vi "删除启动项.vi"(8 "error in (no error)":errorcluster caption="错误输入（无错误）") -> (0 "error out":errorcluster caption="错误输出", 3 "删除标记":bool)   [LabVIEW 2016]
uses:
  <vilib>/registry/registry.llb/Registry RtKey.ctl
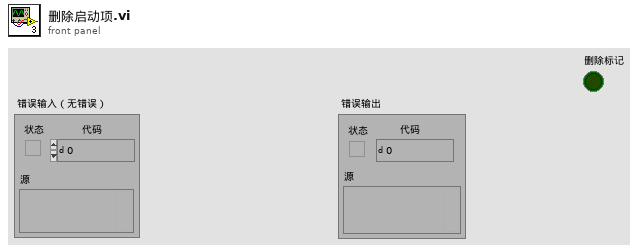
[diagram p1: front panel]
types:
  T1 = typedef "Registry RtKey.ctl" = enum32{"HKEY_CLASSES_ROOT", "HKEY_CURRENT_USER", "HKEY_LOCAL_MACHINE", "HKEY_USERS", "HKEY_PERFORMANCE_DATA", "HKEY_CURRENT_CONFIG", "HKEY_DYN_DATA"}
  T2 = typedef "Registry refnum.ctl" = refnum<k1>
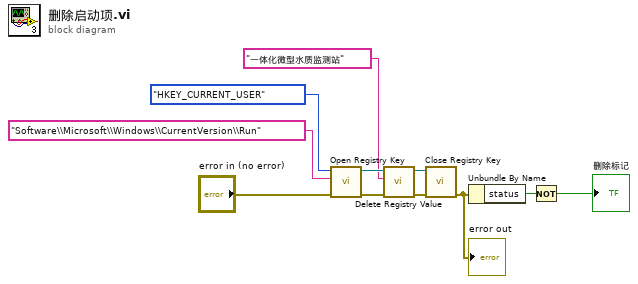
[diagram p0: block diagram]
diagram:
  n1 = call <vilib>:"Open Registry Key.vi"("error in (no error)"="error in (no error)", "subkey"="Software\\Microsoft\\Windows\\CurrentVersion\\Run", "root key (HKEY_LOCAL_MACHINE)"=Registry_RtKey."HKEY_CURRENT_USER") -> ("error out"=w6:errorcluster, "refnum out"=w8:T2)  [unwired: 7 in]
  n2 = call <vilib>:"Delete Registry Value.vi"("error in (no error)"=w6, "value"="一体化微型水质监测站", "refnum"=w8) -> ("error out"=w5:errorcluster, "refnum out"=w7:T2)  [unwired: 7 in]
  n3 = call <vilib>:"Close Registry Key.vi"("error in (no error)"=w5, "refnum"=w7) -> ("error out"=w2:errorcluster)  [unwired: 5 in]
  "error out" <- w2
  n4 = Unbundle By Name(w2) -> ("status"=w1:bool)
  n5 = Not(x=w1) -> (.not. x?=→"删除标记":bool)
